vi "SIM921 Resistance.vi"(10 "Slot":T1(ring), 11 "VISA resource name":refnum<visa-resource-name>) -> (2 "Resistance":dbl[](array[numeric]), 3 "VISA resource name":refnum<visa-resource-name>)   [LabVIEW 2019]
panel:
  out "String Response":string
  out "Error Out":errorcluster
  in  "Error In":errorcluster
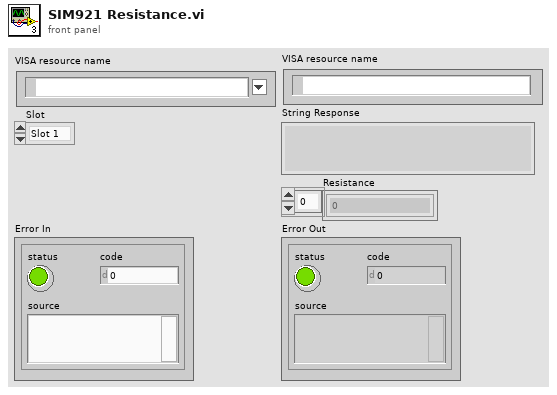
[diagram p1: front panel]
types:
  T1 = enum32{"Slot 1", "Slot 2", "Slot 3", "Slot 4", "Slot 5", "Slot 6", "Slot 7", "Slot 8"}
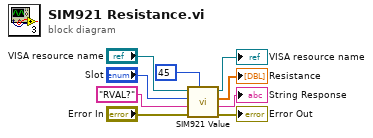
[diagram p0: block diagram]
diagram:
  n1 = call "SIM921 Value.vi"("Wait (ms)"=u32 45, "Error In"="Error In", "Query"="RVAL?" ("format string"), "Slot"="Slot", "VISA resource name"="VISA resource name") -> ("Error Out"=→"Error Out":errorcluster, "String Response"=→"String Response":string, "Resistance"=→"Resistance":dbl[], "VISA resource name"=→"VISA resource name":refnum<visa-resource-name>)  [unwired: 3 in]
